vi "Read ActorStop User Event.vi"(8 "error in (no error)":errorcluster, 11 "eActor in":refnum<class "eActor.lvclass">) -> (0 "error out":errorcluster, 2 "ActorStop":refnum<user-event>, 3 "eActor out":refnum<class "eActor.lvclass">)   [LabVIEW 2015, in "AMS UI.lvlib" / "eActor.lvclass"]
uses:
  eActor.lvclass
  eActor.lvclass/eActor.ctl
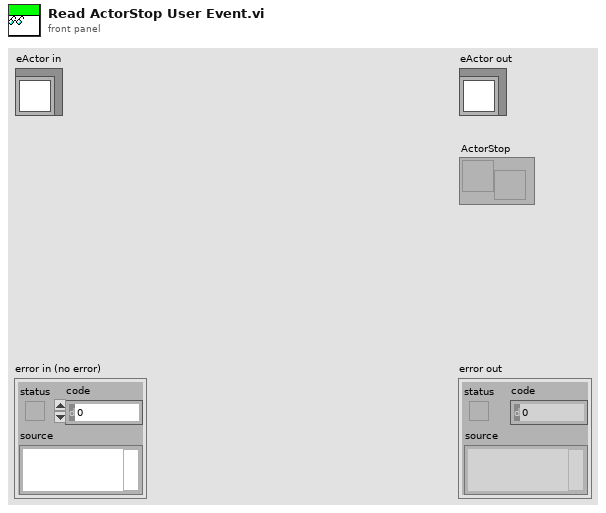
[diagram p1: front panel]
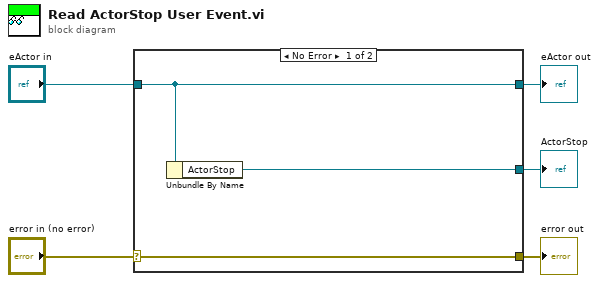
[diagram p0: block diagram]
diagram:
  n1 = case shown="No Error" "error in (no error)" {
    selector: "error in (no error)" -> [w8 w9]
    tunnel: [w8 w9] -> w4
    tunnel: [w7 w10] -> w2
    tunnel: "eActor in" -> [w7 w10]
    tunnel: [w6 _] -> w1
    frame No Error {
      n2 = Unbundle By Name(w7) -> ("ActorStop"=w6:refnum<user-event>)
    }
    frame Error {
    }
  }
  "error out" <- w4
  "eActor out" <- w2
  "ActorStop" <- w1
